vi "NML Action Scripting.vi"() -> ()   [LabVIEW 2024]
uses:
  New NML Data Acq/Sub Controls/Instrument Properties.ctl
  New NML Data Acq/Sub Controls/Public.ctl
  New NML Data Acq/Sub Controls/Private.ctl
  New NML Data Acq/Sub Controls/Instrument Ref.ctl
  New NML Data Acq/Sub Controls/SystemCheckBox-resize.ctl
panel:
  in  "INIT":bool
  out "Data":dbl[](array[numeric]) format="%.4e"
  in  "stop":bool
  in  "Run":bool
  in  "Configure":bool
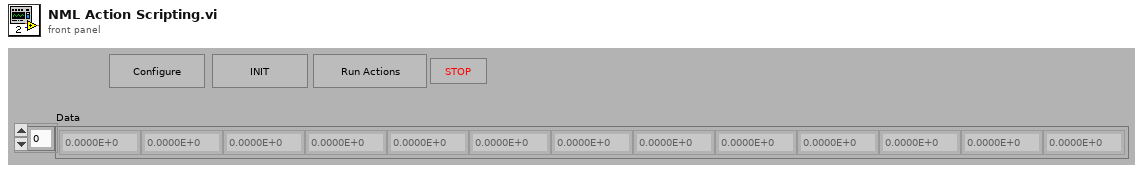
[diagram p1: front panel]
types:
  T1 = typedef "Instrument Properties.ctl" = cluster{"Public":T2, "Private":T3}
  T2 = typedef "Public.ctl" = cluster{"Column Name":string[], "Trace Color":u32[]}
  T3 = typedef "Private.ctl" = cluster{"Path":path, "VI Refnum":T4, "Name":string, "# of Values":i32, "Scale Factors":dbl[], "Display":T5[], "Offset":dbl[]}
  T4 = typedef "Instrument Ref.ctl" = refnum<vi>
  T5 = typedef "SystemCheckBox-resize.ctl" = bool
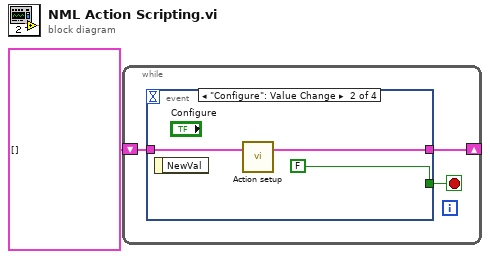
[diagram p0: block diagram]
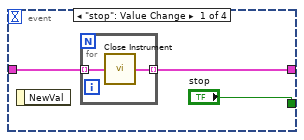
[diagram p2: hidden frame]
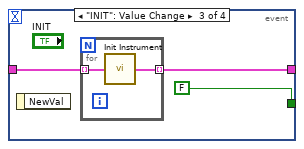
[diagram p3: hidden frame]
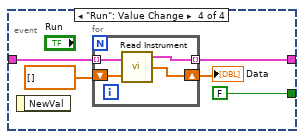
[diagram p4: hidden frame]
diagram:
  n1 = while {
    shift-right: [w3] -> _
    shift-left: T1[] [] ("Setup") -> [w2]
    stop <- w4 stop-if-true
    n2 = event shown="[1] \"Configure\": Value Change" {
      selector: _ -> [_ _ _ _]
      dyn-events: _ -> [_ _ _ _]
      timeout: _ -> [_ _ _ _]
      tunnel: ["stop" FALSE ("stop") FALSE ("stop") FALSE ("stop")] -> w4
      tunnel: w2 -> [w6 w12 w15 w22]
      tunnel: [w5 w11 w14 w21] -> w3
      event "stop": Value Change {
        n3 = event-data() -> ()  [unwired: 1 in, 1 out]
        n4 = for {
          tunnel: w6 -> [w9] mode=indexing
          tunnel: [w8] -> w5 mode=indexing
          n5 = call "Close Instrument.vi"("Instrument Prop"=w9) -> ("Instrument Prop 2"=w8:T1)
        }
      }
      event "Configure": Value Change {
        n6 = event-data() -> ()  [unwired: 1 in, 1 out]
        n7 = call "Action setup.vi"("Setup"=w12) -> ("Array"=w11:T1[])  [unwired: 2 in]
      }
      event "INIT": Value Change {
        n8 = event-data() -> ()  [unwired: 1 in, 1 out]
        n9 = for {
          tunnel: w15 -> [w17] mode=indexing
          tunnel: [w16] -> w14 mode=indexing
          n10 = call "Init Instrument.vi"("Instrument Prop"=w17) -> ("Instrument Prop 2"=w16:T1)
        }
      }
      event "Run": Value Change {
        n11 = event-data() -> ()  [unwired: 1 in, 1 out]
        n12 = for {
          tunnel: w22 -> [w26] mode=indexing
          tunnel: [w25] -> w21 mode=indexing
          shift-right: [w23] -> w19
          shift-left: dbl[] [] ("Array 2") -> [w24]
          n13 = call "Read Instrument.vi"("Instrument Prop"=w26, "Array"=w24) -> ("Instrument Prop 2"=w25:T1, "Array 2"=w23:dbl[])  [unwired: 1 out]
        }
        "Data" <- w19
      }
    }
  }
